vi "Test Serialize Fixed Point.vi"(8 "error in (no error)":errorcluster) -> (0 "error out":errorcluster)   [LabVIEW 2013]
uses:
  src/Serializer/JSON Serializer/JSON Serializer.lvclass
  <vilib>/addons/_JKI Toolkits/Caraya/classes/Test/Test.lvclass
  <vilib>/addons/_JKI Toolkits/Caraya/classes/Assert/Assert.lvclass
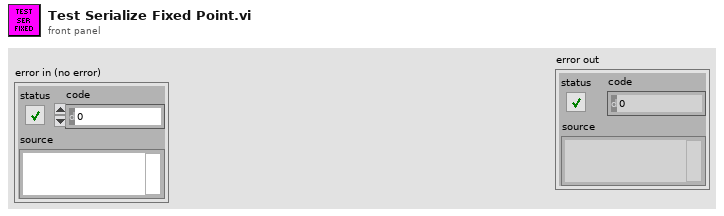
[diagram p1: front panel]
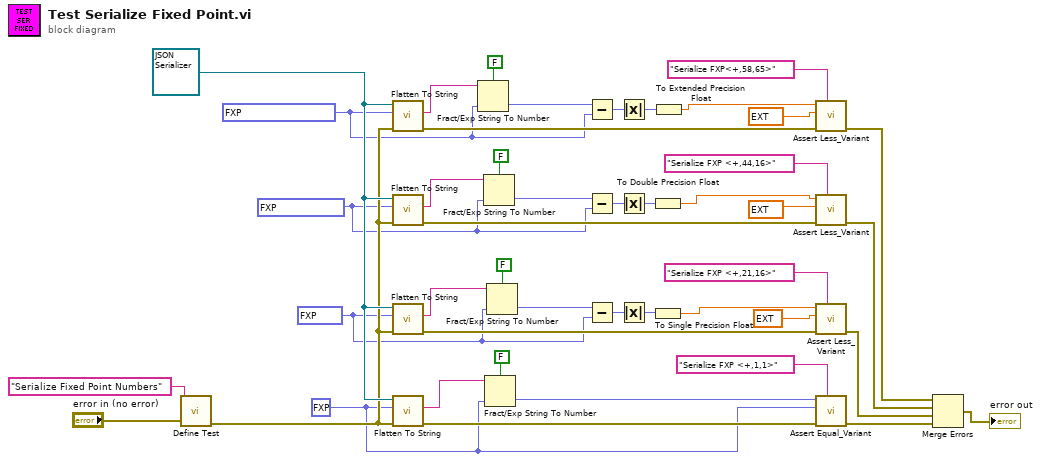
[diagram p0: block diagram]
diagram:
  w36 = refnum<class "JSON Serializer.lvclass"> refnum ("JKI JSON Serialization.lvlib:JSON Serializer.lvclass")
  w10 = fxp<+,1,1> 0.0
  w7 = fxp<+,58,65> dbl? 4.778309726740197e-299
  w9 = fxp<+,21,16> 65529.1875
  w8 = fxp<+,44,16> 42949.67289233953
  n1 = call <vilib>:"Define Test.vi"("error in (no error)"="error in (no error)", "Label (VI Title)"="Serialize Fixed Point Numbers") -> ("error out"=w35:errorcluster)  [unwired: 9 in]
  n2 = call-dynamic "Flatten To String.vi"("error in (no error)"=w35, "Variant"=w7, "JSON Serializer in"=w36) -> ("error out"=w38:errorcluster, "String"=w20:string)  [unwired: 6 in, 1 out]
  n3 = call-dynamic "Flatten To String.vi"("error in (no error)"=w35, "Variant"=w8, "JSON Serializer in"=w36) -> ("error out"=w40:errorcluster, "String"=w22:string)  [unwired: 6 in, 1 out]
  n4 = call-dynamic "Flatten To String.vi"("error in (no error)"=w35, "Variant"=w9, "JSON Serializer in"=w36) -> ("error out"=w42:errorcluster, "String"=w24:string)  [unwired: 6 in, 1 out]
  n5 = call-dynamic "Flatten To String.vi"("error in (no error)"=w35, "Variant"=w10, "JSON Serializer in"=w36) -> ("error out"=w44:errorcluster, "String"=w28:string)  [unwired: 6 in, 1 out]
  n6 = Fract/Exp String To Number(use system decimal point (T)=FALSE, string=w20, default (0 dbl)=w7) -> (number=w18:fxp<+,58,65>)  [unwired: 1 in, 1 out]
  n7 = Fract/Exp String To Number(use system decimal point (T)=FALSE, string=w22, default (0 dbl)=w8) -> (number=w19:fxp<+,44,16>)  [unwired: 1 in, 1 out]
  n8 = Fract/Exp String To Number(use system decimal point (T)=FALSE, string=w28, default (0 dbl)=w10) -> (number=w26:fxp<+,1,1>)  [unwired: 1 in, 1 out]
  n9 = Fract/Exp String To Number(use system decimal point (T)=FALSE, string=w24, default (0 dbl)=w9) -> (number=w17:fxp<+,21,16>)  [unwired: 1 in, 1 out]
  n10 = Subtract(x=w18, y=w7) -> (x-y=w16:fxp<+,64,1>)
  n11 = Subtract(x=w19, y=w8) -> (x-y=w15:fxp<+,1,-27>)
  n12 = Subtract(x=w17, y=w9) -> (x-y=w14:fxp<+,1,-4>)
  n13 = Absolute Value(x=w16) -> (abs(x)=w6:fxp<+,64,1>)
  n14 = Absolute Value(x=w15) -> (abs(x)=w4:fxp<+,1,-27>)
  n15 = Absolute Value(x=w14) -> (abs(x)=w2:fxp<+,1,-4>)
  n16 = To Double Precision Float(number=w4) -> (double precision float=w3:dbl)
  n17 = To Single Precision Float(number=w2) -> (single precision float=w1:sgl)
  n18 = To Extended Precision Float(1:w6) -> (0:w5:ext)
  n19 = call <vilib>:"Assert Less_Variant.vi"("Label"="Serialize FXP<+,58,65>", "error in (no error)"=w38, "Y"=ext 1e-13 ("default (0 DBL)"), "X"=w5) -> ("error out"=w30:errorcluster)  [unwired: 7 in]
  n20 = call <vilib>:"Assert Less_Variant.vi"("Label"="Serialize FXP <+,44,16>", "error in (no error)"=w40, "Y"=ext 1e-11 ("default (0 DBL)"), "X"=w3) -> ("error out"=w31:errorcluster)  [unwired: 7 in]
  n21 = call <vilib>:"Assert Less_Variant.vi"("Label"="Serialize FXP <+,21,16>", "error in (no error)"=w42, "Y"=ext 0.00001 ("default (0 DBL)"), "X"=w1) -> ("error out"=w32:errorcluster)  [unwired: 7 in]
  n22 = call <vilib>:"Assert Equal_Variant.vi"("Label"="Serialize FXP <+,1,1>", "error in (no error)"=w44, "Y"=w10, "X"=w26) -> ("error out"=w33:errorcluster)  [unwired: 7 in]
  n23 = Merge Errors(w30, w31, w32, w33) -> (→"error out":errorcluster)
